vi "CalibrationTest.vi"() -> ()   [LabVIEW 2019]
panel:
  out "Circles Data (calibrated) (Circle Detection 1)":T1(array[cluster])
  in  "Stop Button":bool
  out "Image Out fgv 2":T2(plugin-control)
  out "Image Out fgv":T2(plugin-control)
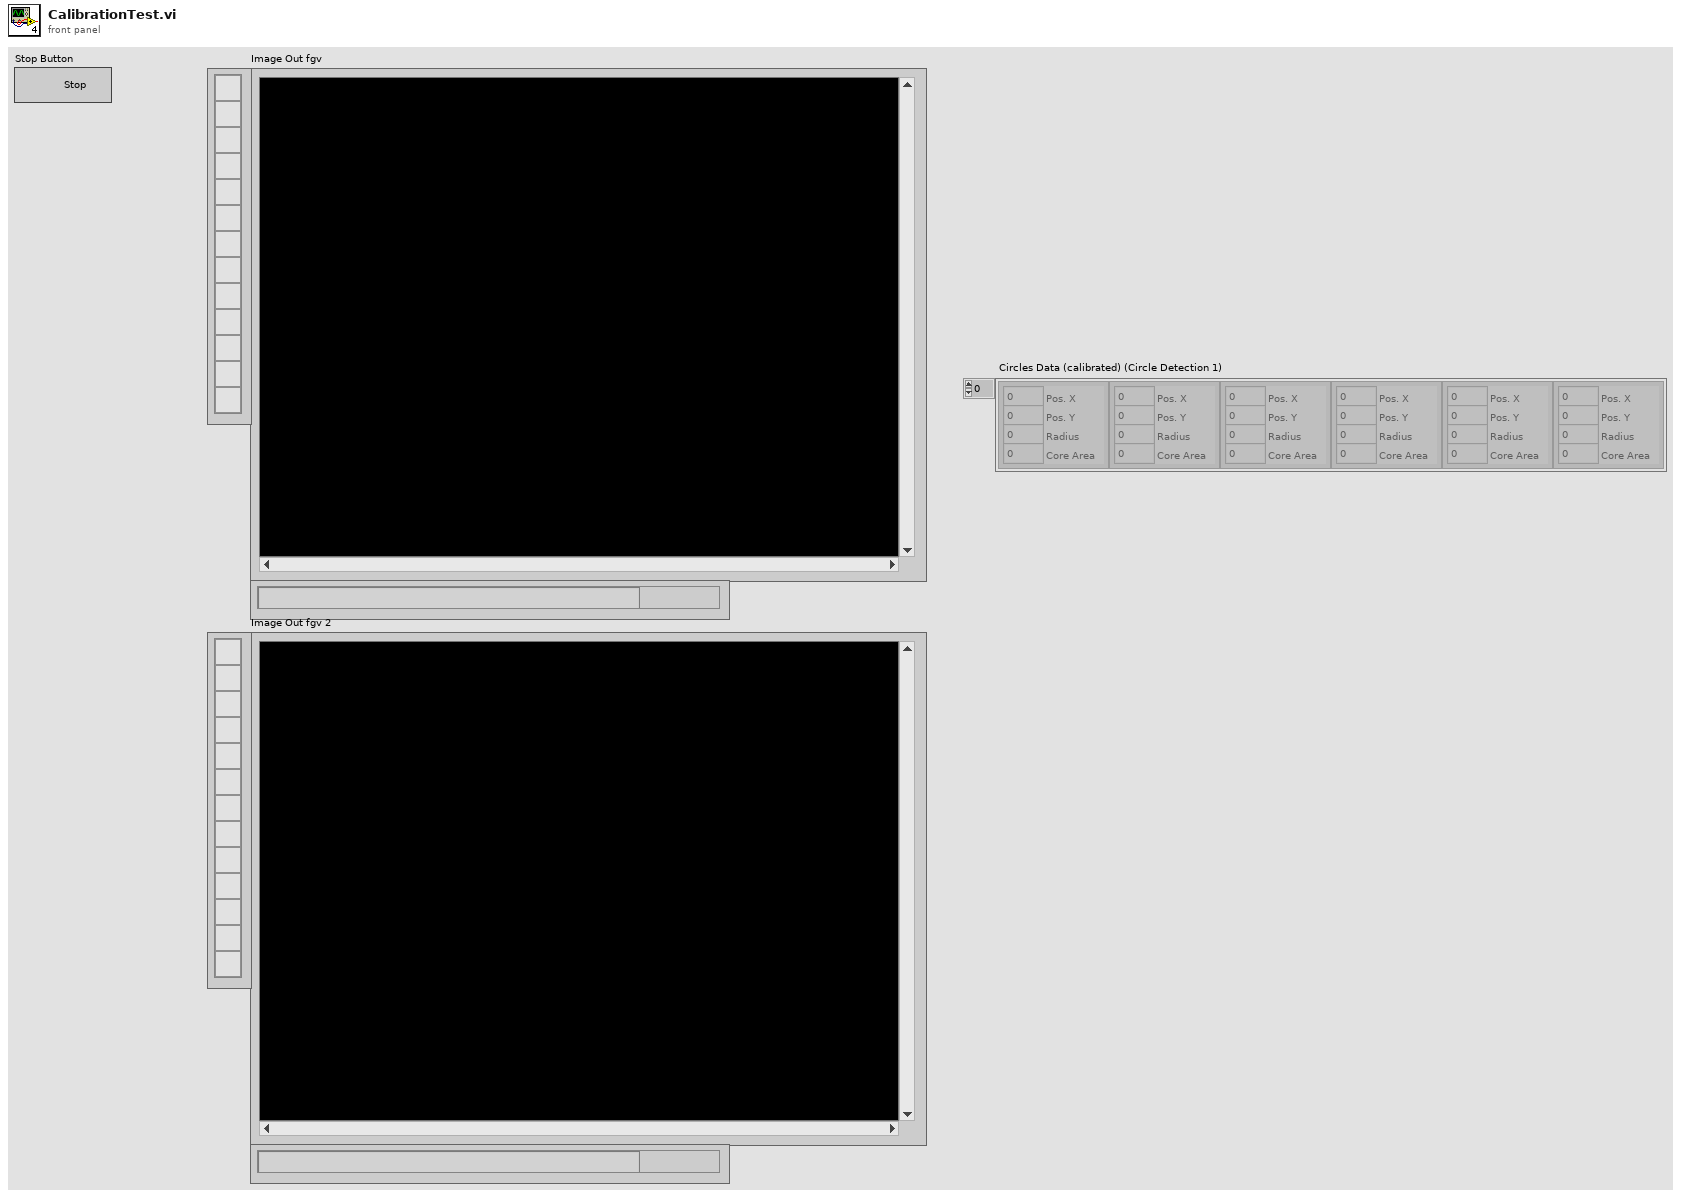
[diagram p1: front panel]
types:
  T1 = cluster{"Pos. X":i32, "Pos. Y":i32, "Radius":i32, "Core Area":i32}[]
  T2 = typedef "IMAQ Image.ctl" = refnum<image>
  T3 = typedef "Image Type" = u32
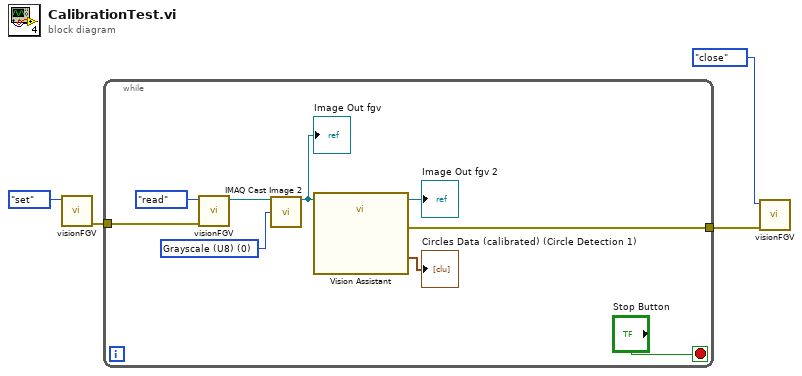
[diagram p0: block diagram]
diagram:
  n1 = call "visionFGV.vi"("Function"=enum16{"set", "read", "close"}."set") -> ("error out"=w4:errorcluster)  [unwired: 9 in, 1 out]
  n2 = while {
    tunnel: w4 -> [w12]
    tunnel: [w9] -> w2
    stop <- "Stop Button" stop-if-true
    w7 = T3 0 items=["Grayscale (U8)", "Grayscale (I16)", "Grayscale (SGL)", "Complex (CSG)", "RGB (U32)", "HSL (U32)", "RGB (U64)", "Grayscale (U16)"] ("Image Type")
    n3 = call "visionFGV.vi"("Error In"=w12, "Function"=enum16{"set", "read", "close"}."read") -> ("Image Out fgv"=w8:T2)  [unwired: 8 in, 1 out]
    n4 = call "IMAQ Cast Image 2"("Image Src"=w8, "Image Type"=w7) -> ("Image Dst Out"=w6:T2)  [unwired: 12 in, 1 out]
    "Image Out fgv" <- w6
    n5 = call "Vision Assistant"("Image In"=w6) -> ("Image Out"=→"Image Out fgv 2":T2, "Circles Data (calibrated) (Circle Detection 1)"=→"Circles Data (calibrated) (Circle Detection 1)":T1, "error out"=w9:errorcluster)  [unwired: 24 in]
  }
  n6 = call "visionFGV.vi"("Error In"=w2, "Function"=enum16{"set", "read", "close"}."close") -> ()  [unwired: 8 in, 2 out]
